vi "termoSim.vi"() -> ()   [LabVIEW 2015]
panel:
  out "Waveform Chart":dbl(graph)
  out "String":string
  in  "stop":bool
  out "Thermometer":dbl(slide) scale=0.0..100.0
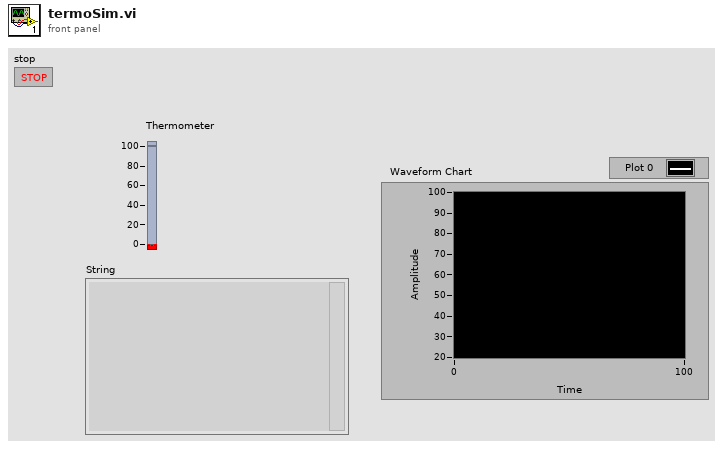
[diagram p1: front panel]
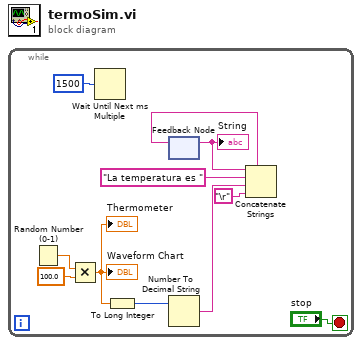
[diagram p0: block diagram]
diagram:
  n1 = while {
    stop <- "stop" stop-if-true
    n2 = Random Number (0-1)() -> (number: 0 to 1=w11:dbl)
    n3 = Multiply(x=w11, y=100.0) -> (x*y=w2:dbl)
    "Thermometer" <- w2
    "Waveform Chart" <- w2
    n4 = Wait Until Next ms Multiple(millisecond multiple=u32 1500 ("millisecond timer value")) -> ()  [unwired: 1 out]
    n5 = To Long Integer(number=w2) -> (32bit integer=w1:i32)
    n6 = feedback #1() -> (w3:string)  [unwired: 1 in]
    "String" <- w3
    n7 = Number To Decimal String(number=w1) -> (decimal integer string=w8:string)  [unwired: 1 in]
    n8 = Concatenate Strings(w3, "La temperatura es ", w8, "\r") -> (w5:string)
    n9 = feedback-in #1(w5) -> ()
  }
